vi "PID Set Points.vi"() -> ()   [LabVIEW 2011]
panel:
  in  "Shooter Enabled":bool
  out "Hood Voltage":dbl
  out "ShooterSet Speed":dbl
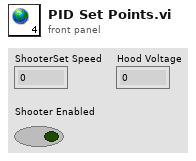
[diagram p1: front panel]
diagram:
